vi "Breakdown ROI to miniscans.vi"(11 "ROI Attributes":T1[](array[typedef]) {"Apparent Frame Size" format="%#_6f"; "Original FOV (um)" format="%#_6f"; "Pixels per miniscan" format="%#_6f"; "Dwell Time per pixel" format="%#_6f"; "Resolution" format="%#_6f"; "ROI group ID" format="%#_6f"; "Laser Power (%)" format="%#_6f"; "Zoom" format="%#_6f"; "Frame Size" format="%#_6f"; "Number of lines" format="%#_6f"; "Composite ID" format="%#_6f"; "Angle (deg)" format="%#_6f"; "ROI Time (ns)" format="%#_6f"; "ROI ID" format="%#_6f"; "Pixels in ROI" format="%#_6f"; "ROI index" format="%#_6f"; "Z stop" format="%#_6f"; "Y stop" format="%#_6f"; "X stop" format="%#_6f"; "Z start" format="%#_6f"; "X start" format="%#_6f"; "Y start" format="%#_6f"}) -> (1 "Laser(V)":dbl[](array[numeric]), 3 "ROI Attributes (broken down to miniscans)":T1[](array[typedef]) {"Apparent Frame Size" format="%#_6f"; "Original FOV (um)" format="%#_6f"; "Pixels per miniscan" format="%#_6f"; "Dwell Time per pixel" format="%#_6f"; "Resolution" format="%#_6f"; "ROI group ID" format="%#_6f"; "Laser Power (%)" format="%#_6f"; "Zoom" format="%#_6f"; "Frame Size" format="%#_6f"; "Number of lines" format="%#_6f"; "Composite ID" format="%#_6f"; "Angle (deg)" format="%#_6f"; "ROI Time (ns)" format="%#_6f"; "ROI ID" format="%#_6f"; "Pixels in ROI" format="%#_6f"; "ROI index" format="%#_6f"; "Z stop" format="%#_6f"; "Y stop" format="%#_6f"; "X stop" format="%#_6f"; "Z start" format="%#_6f"; "X start" format="%#_6f"; "Y start" format="%#_6f"})   [LabVIEW 2020]
uses:
  User Interface/Visualisation/Functional Imaging Viewer/Typedefs/ROI parameters data type.ctl
  Global Variables/General Globals.vi
panel:
  out "logical AND":bool
  out "Output size":i32
  out "Input size":i32
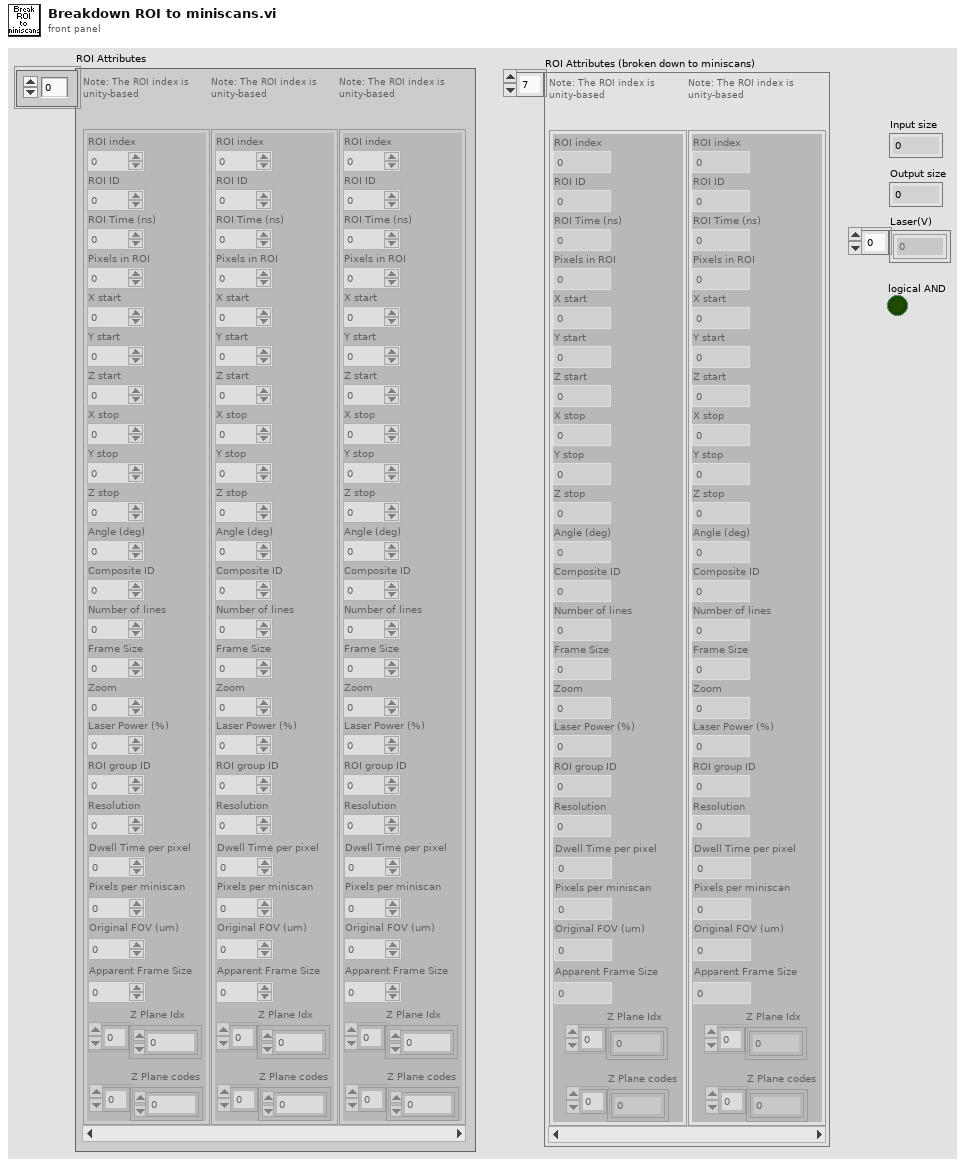
[diagram p1: front panel]
types:
  T1 = typedef "ROI parameters data type.ctl" = cluster{"ROI index":dbl, "ROI ID":dbl, "ROI Time (ns)":dbl, "Pixels in ROI":dbl, "X start":dbl, "Y start":dbl, "Z start":dbl, "X stop":dbl, "Y stop":dbl, "Z stop":dbl, "Angle (deg)":dbl, "Composite ID":dbl, "Number of lines":dbl, "Frame Size":dbl, "Zoom":dbl, "Laser Power (%)":dbl, "ROI group ID":dbl, "Resolution":dbl, "Dwell Time per pixel":dbl, "Pixels per miniscan":dbl, "Original FOV (um)":dbl, "Apparent Frame Size":dbl, "Z Plane Idx":i32[], "Z Plane codes":i32[]}
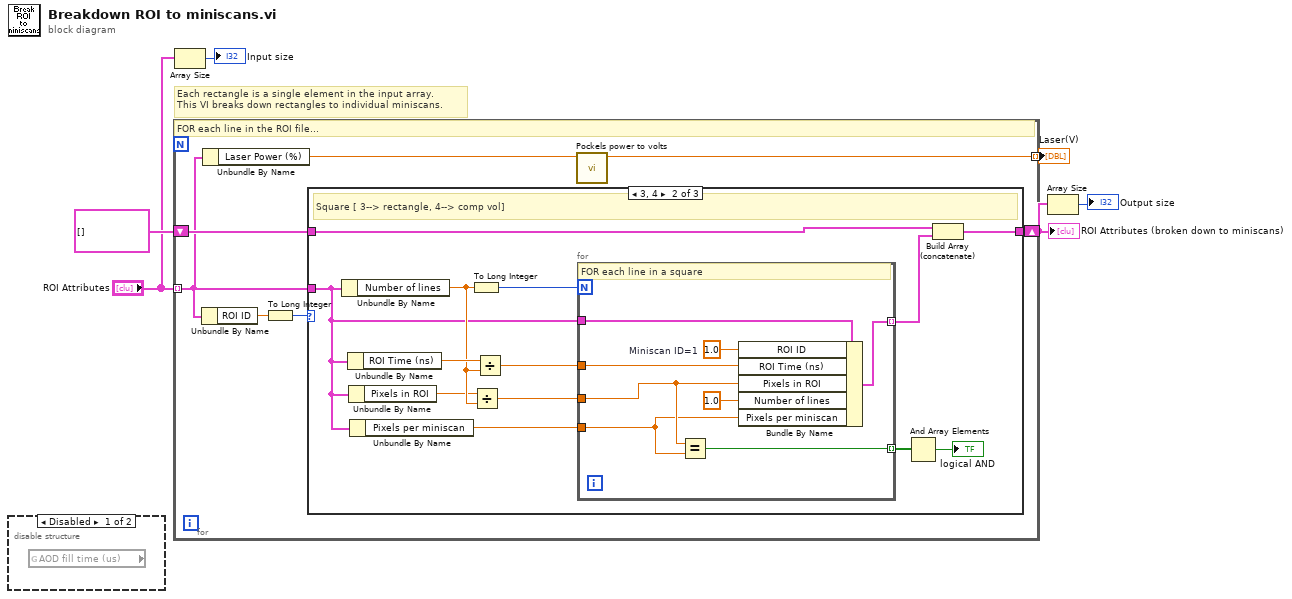
[diagram p0: block diagram]
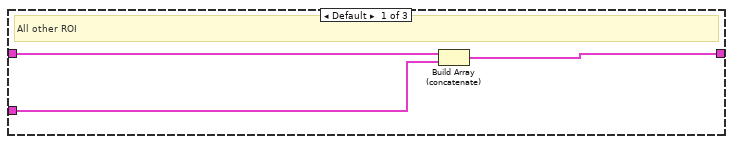
[diagram p3: hidden frame]
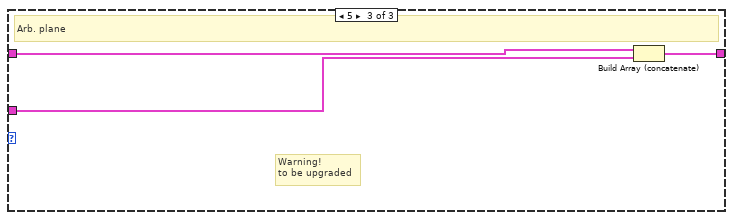
[diagram p4: hidden frame]
diagram:
  # "Each rectangle is a single element in the input array.\nThis VI breaks down rectangles to individual miniscans."
  n1 = disable-structure shown="Disabled" {
    frame Disabled {
      n2 = global read "General Globals.vi" "AOD fill time (us)"() -> ()  [unwired: 1 out]
    }
    frame Enabled {
    }
  }
  n3 = for {
    tunnel: "ROI Attributes" -> [w9] mode=indexing
    shift-right: [w10] -> w2
    shift-left: T1[] [] ("ROI Coordinates (broken down to miniscans)") -> [w11]
    tunnel: [w7] -> w1 mode=indexing
    # "FOR each line in the ROI file..."
    n4 = Unbundle By Name(w9) -> ("ROI ID"=w13:dbl)
    n5 = Unbundle By Name(w9) -> ("Laser Power (%)"=w8:dbl)
    n6 = To Long Integer(number=w13) -> (32bit integer=w12:i32)
    n7 = case shown="3, 4" w12 {
      tunnel: w9 -> [w15 w20 w38]
      tunnel: [w14 w28 w40] -> w10
      tunnel: w11 -> [w16 w27 w39]
      frame Default {
        # "All other ROI"
        n8 = Build Array (concatenate)(w16, w15) -> (w14:T1[])
      }
      frame 3, 4 {
        # "Square [ 3--> rectangle, 4--> comp vol]"
        n9 = Unbundle By Name(w20) -> ("Number of lines"=w24:dbl)
        n10 = Unbundle By Name(w20) -> ("ROI Time (ns)"=w26:dbl)
        n11 = Unbundle By Name(w20) -> ("Pixels in ROI"=w23:dbl)
        n12 = Unbundle By Name(w20) -> ("Pixels per miniscan"=w19:dbl)
        n13 = To Long Integer(number=w24) -> (32bit integer=w25:i32)
        n14 = Divide(x=w23, y=w24) -> (x/y=w22:dbl)
        n15 = Divide(x=w26, y=w24) -> (x/y=w21:dbl)
        n16 = for {
          N: w25 -> [_]
          tunnel: w20 -> [w37]
          tunnel: [w36] -> w29 mode=indexing
          tunnel: w21 -> [w34]
          tunnel: w22 -> [w32]
          tunnel: w19 -> [w31]
          tunnel: [w30] -> w18 mode=indexing
          w35 = 1.0  # Miniscan ID=1
          # "FOR each line in a square"
          n17 = Equal?(x=w32, y=w31) -> (x = y?=w30:bool)
          n18 = Bundle By Name(cluster=w37, "ROI ID"=w35, "ROI Time (ns)"=w34, "Pixels in ROI"=w32, "Number of lines"=1.0, "Pixels per miniscan"=w31) -> (w36:T1)
        }
        n19 = And Array Elements(Boolean array=w18) -> (logical AND=→"logical AND":bool)
        n20 = Build Array (concatenate)(w27, w29) -> (w28:T1[])
      }
      frame 5 {
        # "Warning!\nto be upgraded"
        # "Arb. plane"
        n21 = Build Array (concatenate)(w39, w38) -> (w40:T1[])
      }
    }
    n22 = call "Pockels power to volts.vi"("Pockels power (%)"=w8) -> ("Pockels control voltage (V)"=w7:dbl)  [unwired: 8 in, 2 out]
  }
  "ROI Attributes (broken down to miniscans)" <- w2
  "Laser(V)" <- w1
  n23 = Array Size(array="ROI Attributes") -> (size(s)=→"Input size":i32)
  n24 = Array Size(array=w2) -> (size(s)=→"Output size":i32)
